vi "MU Calibration Preconfigure Number Of Master Periods.vi"(8 "error in (no error)":errorcluster, 10 "NumberOfMasterPeriods (0=autodetect)":u32, 11 "calibration":T1) -> (0 "error out":errorcluster, 3 "Return value":bool)   [LabVIEW 2017, in "MU_3SL_interface.lvlib"]
uses:
  MU_3SL_interface.lvlib
  handles/CalibrationHandle.ctl
  lib/MU_3SL_interface.dll
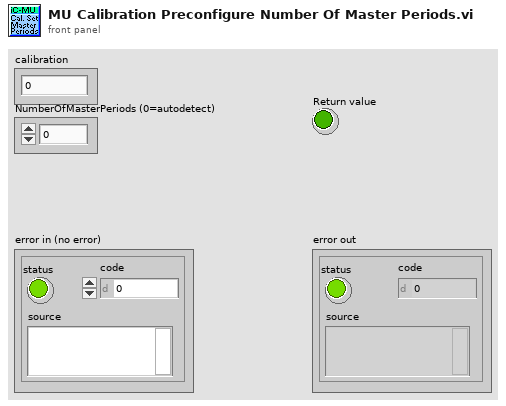
[diagram p1: front panel]
types:
  T1 = typedef "MU_3SL_interface.lvlib/CalibrationHandle.ctl" = u64
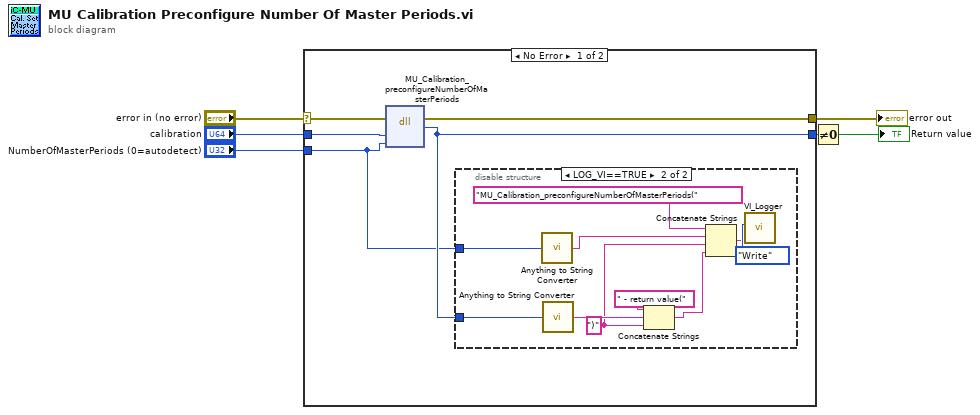
[diagram p0: block diagram]
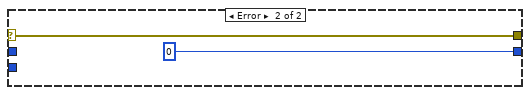
[diagram p3: hidden frame]
diagram:
  n1 = case shown="No Error" "error in (no error)" {
    selector: "error in (no error)" -> [w11 w23]
    tunnel: [w9 u32 0 ("return type")] -> w2
    tunnel: [w8 w23] -> w6
    tunnel: "calibration" -> [w10 _]
    tunnel: "NumberOfMasterPeriods (0=autodetect)" -> [w7 _]
    frame No Error {
      n2 = dll-call lib="C:/Users/bes/AppData/Roaming/work/mu_9so/icsubmodules/soft_mu_3sl_master/lv_interface/lib/MU_3SL_interface**.*" fn="MU_Calibration_preconfigureNumberOfMasterPeriods"(error in=w11, "calibration"=w10, "NumberOfMasterPeriods"=w7) -> (error out=w8:errorcluster, "return type"=w9:u8)  [unwired: 4 in, 1 out]
      n3 = disable-structure shown="LOG_VI==TRUE" {
        disable-tunnel: w9 -> [_ w17]
        disable-tunnel: w7 -> [_ w15]
        frame condition #0 {
        }
        frame condition #1 (active) {
          w13 = ")" ("string")
          n4 = call "Anything to String Converter.vi"("anything"=w15) -> ("String"=w14:string)
          n5 = call "Anything to String Converter.vi"("anything"=w17) -> ("String"=w16:string)
          n6 = Concatenate Strings(" - return value(" ("string"), w16, w13) -> (w12:string)
          n7 = Concatenate Strings("MU_Calibration_preconfigureNumberOfMasterPeriods(" ("Info in"), w14, w13, w12) -> (w19:string)
          n8 = call "VI_Logger.vi"("Action (Read)"=enum16{"Write", "Read"}."Write", "Info in"=w19) -> ()  [unwired: 8 in, 2 out]
        }
      }
    }
    frame Error {
    }
  }
  "error out" <- w6
  n9 = Not Equal To 0?(x=w2) -> (x != 0?=→"Return value":bool)
